vi "Parse Inverter Data.vi"(8 "error in (no error)":errorcluster, 10 "Inverter  ERD Data":T3[](array[typedef]) {"ERD Number" format="%.0x"}, 11 "GEA3 ERD Data Out":T1) -> (0 "error out":errorcluster, 2 "ERD Data Output":T1, 3 "Inverter Data String":string[][](array[string]))   [LabVIEW 2020]
uses:
  Water Heating Specific/Type Definitions/GEA3 HEWH ERD Data.ctl
  Water Heating Specific/Type Definitions/GEA3 HEWH Mixing Valve.ctl
  type defs/ERD Read Data Out.ctl
  library/GEA2_Toolkit.lvlib
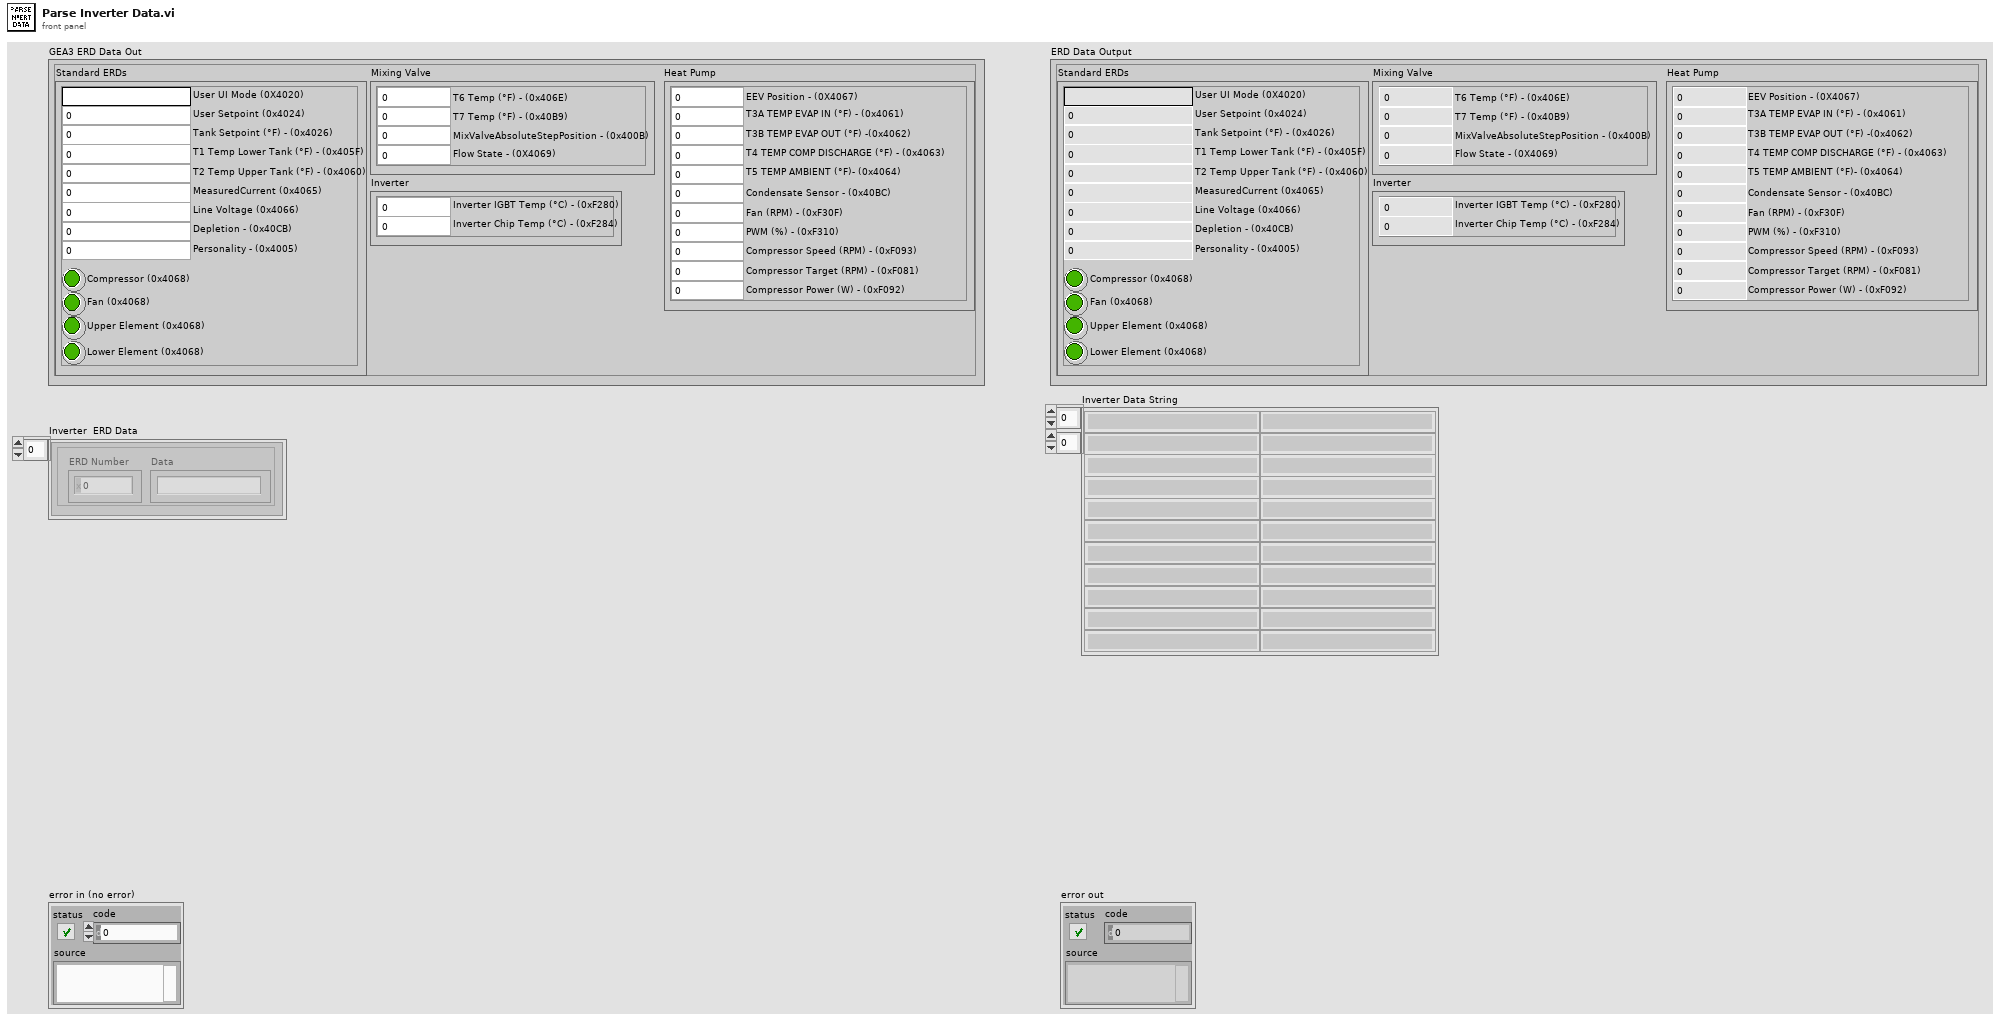
[diagram p1: front panel]
types:
  T1 = typedef "GEA3 HEWH ERD Data.ctl" = cluster{"Mixing Valve":T2, "Standard ERDs":cluster{"User UI Mode (0X4020)":string, "User Setpoint (0x4024)":u16, "Compressor (0x4068)":bool, "Lower Element (0x4068)":bool, "Upper Element (0x4068)":bool, "Fan (0x4068)":bool, "T1 Temp Lower Tank (°F) - (0x405F)":dbl, "T2 Temp Upper Tank (°F) - (0x4060)":dbl, "Line Voltage (0x4066)":u16, "MeasuredCurrent (0x4065)":dbl, "Tank Setpoint (°F) - (0x4026)":u16, "Depletion - (0x40CB)":u16, "Personality - (0x4005)":u16}, "Heat Pump":cluster{"EEV Position - (0X4067)":u16, "T3A TEMP EVAP IN (°F) - (0x4061)":dbl, "T3B TEMP EVAP OUT (°F) -(0x4062)":dbl, "T4 TEMP COMP DISCHARGE (°F) - (0x4063)":dbl, "T5 TEMP AMBIENT (°F)- (0x4064)":dbl, "Condensate Sensor - (0x40BC)":u16, "Fan (RPM) - (0xF30F)":u16, "PWM (%) - (0xF310)":u16, "Compressor Speed (RPM) - (0xF093)":u16, "Compressor Target (RPM) - (0xF081)":u16, "Compressor Power (W) - (0xF092)":u16}, "Inverter":cluster{"Inverter IGBT Temp (°C) - (0xF280)":dbl, "Inverter Chip Temp (°C) - (0xF284)":dbl}}
  T2 = typedef "GEA3 HEWH Mixing Valve.ctl" = cluster{"T7 Temp (°F) - (0x40B9)":dbl, "MixValveAbsoluteStepPosition - (0x400B)":i16, "Flow State - (0X4069)":u8, "T6 Temp (°F) - (0x406E)":dbl}
  T3 = typedef "GEA2_Toolkit.lvlib/ERD Read Data Out.ctl" = cluster{"ERD Number":u16, "Data":string}
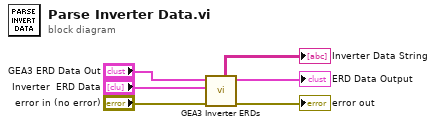
[diagram p0: block diagram]
diagram:
  n1 = call "GEA3 Inverter ERDs.vi"("error in"="error in (no error)", "Inverter  ERD Data"="Inverter  ERD Data", "ERD Data"="GEA3 ERD Data Out") -> ("error out"=→"error out":errorcluster, "ERD Data Output"=→"ERD Data Output":T1, "Inverter Data"=→"Inverter Data String":string[][])  [unwired: 6 in]
